vi "closeAllXML.vi"(8 "error in (no error)":errorcluster, 11 "NativeXML in":refnum<class "NativeXML.lvclass">) -> (0 "error out":errorcluster)   [LabVIEW 2011, in "Tools.lvlib" / "xml.lvlib" / "NativeXML.lvclass"]
uses:
  NativeXML.lvclass
  NativeXML.lvclass/NativeXML.ctl
  <vilib>/xml/Close Reference(Node).vi
  <vilib>/xml/NI_XML.lvlib
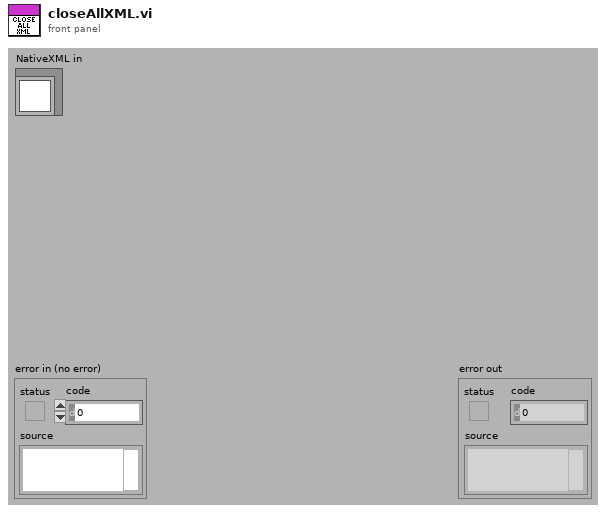
[diagram p1: front panel]
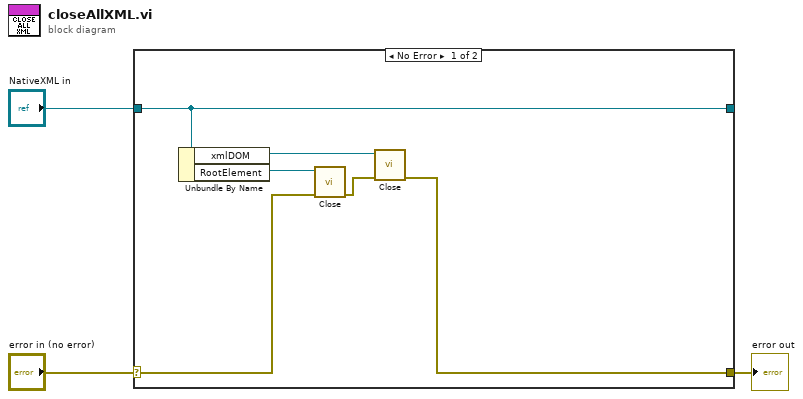
[diagram p0: block diagram]
diagram:
  n1 = case shown="No Error" "error in (no error)" {
    selector: "error in (no error)" -> [w7 w11]
    tunnel: [w4 w11] -> w2
    tunnel: [w9 w10] -> _
    tunnel: "NativeXML in" -> [w9 w10]
    frame No Error {
      n2 = Unbundle By Name(w9) -> ("xmlDOM"=w5:refnum<k20>, "RootElement"=w8:refnum<k20>)
      n3 = call-poly <vilib>:"Close.vi"("error in (no error)"=w7, "node"=w8) -> ("error out"=w6:errorcluster)  [unwired: 7 in]
      n4 = call-poly <vilib>:"Close.vi"("error in (no error)"=w6, "node"=w5) -> ("error out"=w4:errorcluster)  [unwired: 7 in]
    }
    frame Error {
    }
  }
  "error out" <- w2
